vi "niDTS BT INSTR TX WaitOnIdle.vi"(8 "error in (no error)":errorcluster, 9 "Result Instance":i32=1, 10 "Driver Instance":i32=1, 11 "niDTS BT INSTR TX in":refnum<class "niDTS BT INSTR TX.lvclass">) -> (0 "error out":errorcluster, 3 "niDTS BT INSTR TX out":refnum<class "niDTS BT INSTR TX.lvclass">)   [LabVIEW 2015, in "niDTS BT.lvlib" / "niDTS BT INSTR TX.lvclass"]
uses:
  niDTS BT INSTR TX.lvclass
  niDTS BT INSTR TX.lvclass/niDTS BT INSTR TX.ctl
  RiviInstDriver/InstDriver/Objects/InstDriver.lvclass
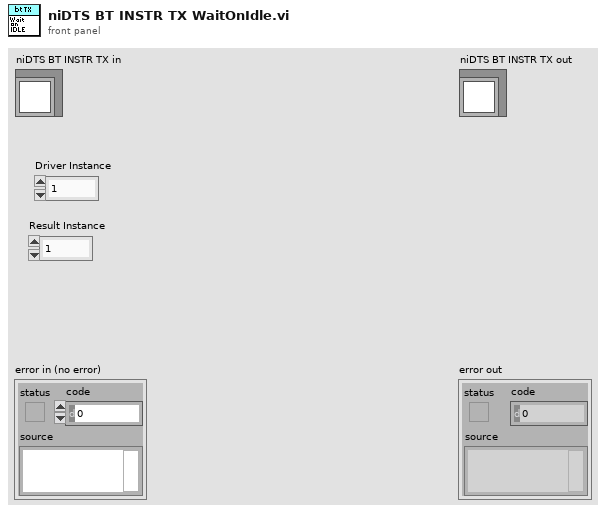
[diagram p1: front panel]
types:
  T1 = typedef "niRfsaBT.lvclass/niRfsaBT INC Handle.ctl" = refnum<data-value>
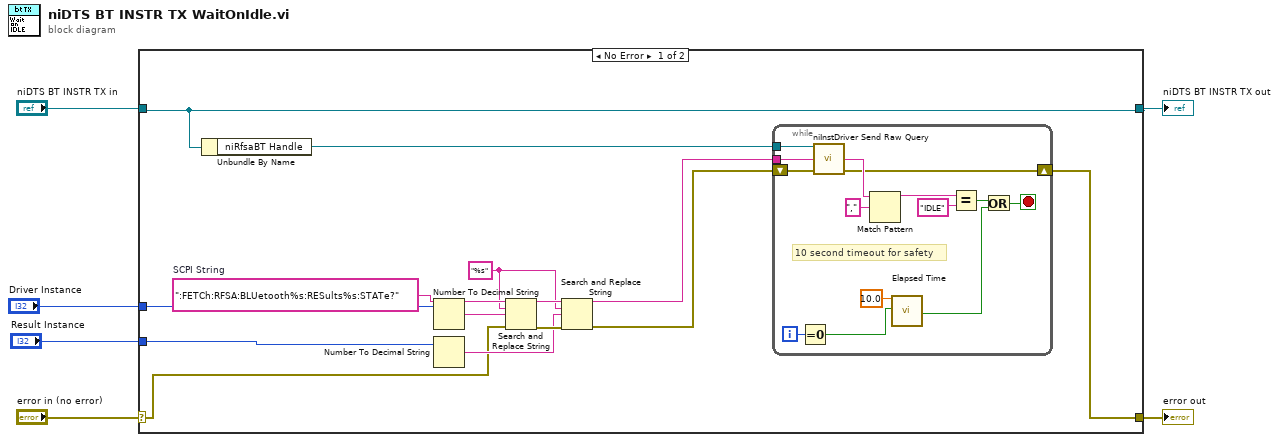
[diagram p0: block diagram]
diagram:
  n1 = case shown="No Error" "error in (no error)" {
    selector: "error in (no error)" -> [w8 w36]
    tunnel: [w7 w36] -> w5
    tunnel: [w11 w35] -> w3
    tunnel: "niDTS BT INSTR TX in" -> [w11 w35]
    tunnel: "Driver Instance" -> [w10 _]
    tunnel: "Result Instance" -> [w9 _]
    frame No Error {
      w15 = "%s" ("search string")
      w17 = ":FETCh:RFSA:BLUetooth%s:RESults%s:STATe?"  # SCPI String
      n2 = Unbundle By Name(w11) -> ("niRfsaBT Handle"=w18:T1)
      n3 = Number To Decimal String(number=w10) -> (decimal integer string=w13:string)  [unwired: 1 in]
      n4 = Number To Decimal String(number=w9) -> (decimal integer string=w12:string)  [unwired: 1 in]
      n5 = Search and Replace String(input string=w17, search string=w15, replace string=w13, error in=w8) -> (result string=w16:string, error out=w14:errorcluster)  [unwired: 4 in, 2 out]
      n6 = Search and Replace String(input string=w16, search string=w15, replace string=w12, error in=w14) -> (result string=w19:string, error out=w20:errorcluster)  [unwired: 4 in, 2 out]
      n7 = while {
        tunnel: w18 -> [w34]
        tunnel: w19 -> [w33]
        shift-right: [w21] -> w7
        shift-left: w20 -> [w32]
        i -> [w25]
        stop <- w26 stop-if-true
        # "10 second timeout for safety"
        n8 = Equal To 0?(x=w25) -> (x = 0?=w24:bool)
        n9 = call "niInstDriver Send Raw Query.vi"("InstDriver Handle in"=w34, "Query"=w33, "error in (no error)"=w32) -> ("Response"=w28:string, "error out"=w21:errorcluster)  [unwired: 10 in, 1 out]
        n10 = Match Pattern(string=w28, regular expression=",") -> (before substring=w30:string)  [unwired: 1 in, 3 out]
        n11 = call "Elapsed Time"("Time Target (s)"=10.0, "Reset"=w24) -> ("Time has Elapsed"=w22:bool)  [unwired: 10 in, 7 out]
        n12 = Equal?(x=w30, y="IDLE") -> (x = y?=w27:bool)
        n13 = Or(x=w27, y=w22) -> (x .or. y?=w26:bool)
      }
    }
    frame Error {
    }
  }
  "error out" <- w5
  "niDTS BT INSTR TX out" <- w3
